vi "Monitor Stream.vi"(8 "error in (no error)":errorcluster, 10 "Refnum in":refnum<k20>[](array[refnum]), 11 "2 USRPs?":bool[](array[boolean])) -> (0 "error out":errorcluster, 2 "Samples Transferred":u64[](array[numeric]), 3 "Stream State":T1[](array[typedef]))   [LabVIEW 2016]
uses:
  <instrlib>/_niInstr/Streaming/v1/Common/Stream State.ctl
  <vilib>/Utility/error.llb/Error Cluster From Error Code.vi
  <vilib>/ErrorRing/Error Ring.xnode
  <instrlib>/_niInstr/Streaming/v1/Host/niInstr Streaming v1 Host.lvlib
  <instrlib>/_niInstr/Streaming/v1/Common/niInstr Streaming v1 Common.lvlib
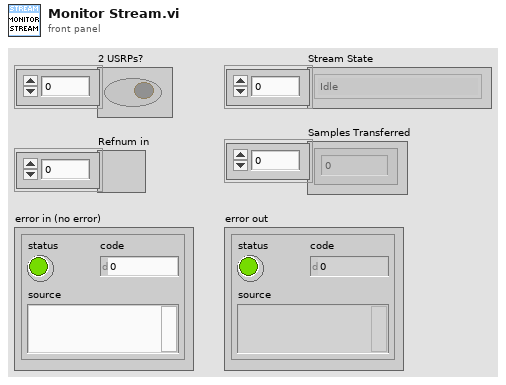
[diagram p1: front panel]
types:
  T1 = typedef "niInstr Streaming v1 Common.lvlib/Stream State.ctl" = enum8{"Idle", "Finite Transfer", "Continuous", "Done", "Error", "Not Ready", "Cancel"}
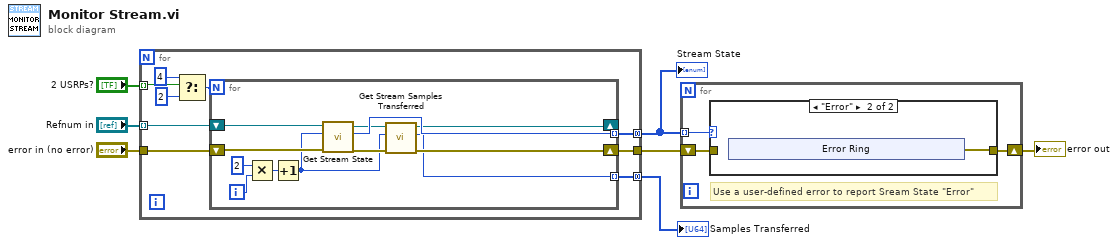
[diagram p0: block diagram]
diagram:
  n1 = for {
    tunnel: "error in (no error)" -> [w16]
    tunnel: "Refnum in" -> [w15] mode=indexing
    tunnel: [w14] -> w2
    tunnel: "2 USRPs?" -> [w10] mode=indexing
    tunnel: [w9] -> w6 mode=concatenating
    tunnel: [w8] -> w3 mode=concatenating
    n2 = Select(t=4, s=w10, f=2) -> (s? t:f=w11:i32)
    n3 = for {
      N: w11 -> [_]
      tunnel: [w26] -> w8 mode=indexing
      shift-right: [w18] -> _
      shift-left: w15 -> [w28]
      shift-right: [w21] -> w14
      shift-left: w16 -> [w27]
      tunnel: [w20] -> w9 mode=indexing
      i -> [w23]
      n4 = Multiply(x=2, y=w23) -> (x*y=w25:i32)
      n5 = Increment(x=w25) -> (x+1=w17:i32)
      n6 = call <instrlib>:"Get Stream State.vi"("error in (no error)"=w27, "stream index"=w17, "refnum in"=w28) -> ("error out"=w22:errorcluster, "stream state"=w26:T1, "refnum out"=w19:refnum<k20>)  [unwired: 6 in]
      n7 = call <instrlib>:"Get Stream Samples Transferred.vi"("error in (no error)"=w22, "stream index"=w17, "refnum in"=w19) -> ("error out"=w21:errorcluster, "samples transferred"=w20:u64, "refnum out"=w18:refnum<k20>)  [unwired: 6 in]
    }
  }
  "Stream State" <- w3
  "Samples Transferred" <- w6
  n8 = for {
    tunnel: w3 -> [w31] mode=indexing
    shift-right: [w29] -> w1
    shift-left: w2 -> [w30]
    # "Use a user-defined error to report Sream State \"Error\""
    n9 = case shown="\"Error\"" w31 {
      tunnel: w30 -> [w32 _]
      tunnel: [w32 w33] -> w29
      frame "Idle", Default {
      }
      frame "Error" {
        n10 = xnode "Error Ring"() -> ("error out"=w33:errorcluster)
      }
    }
  }
  "error out" <- w1
